vi "JTAG Clocks.vi"(0 "Adjust MCLK":bool, 1 "MCLK Source":u8(ring) items=["DCOCLK", "DCOCLK", "XT2CLK", "LFXT1/VLOCLK"], 2 "MCLK Divider":u8(ring) items=["1", "2", "4", "8"], 3 "Adjust SMCLK":bool, 4 "SMCLK Source":u8(ring) items=["DCOCLK", "XT2/LFXT1/VLOCLK"], 5 "SMCLK Divider":u8(ring) items=["1", "2", "4", "8"], 7 "error in (no error)":errorcluster, 8 "Adjust ACLK":bool, 9 "Adjust DCOCLK":bool, 10 "ACLK Source":u8(ring) items=["LFXT1CLK", "Reserved", "VLOCLK", "DIG EXT CLK"], 11 "DCO Range[0-15]":u8 max=15 step=1, 12 "ACLK Divider":u8(ring) items=["1", "2", "4", "8"], 13 "DCO Select[0-7]":u8 max=7 step=1, 15 "DCO Mod[0-31]":u8 max=31 step=1, 22 "DCO Ext. Res.":bool, 23 "LFXT1 XTS \"HI\"":bool, 24 "LFXT1 CAP":u8(ring)=1 items=["1pF", "6pF", "10pF", "12.5pF"], 25 "XT2 \"OFF\"":bool) -> (20 "LFXT1 Fault":bool, 21 "XT2 Fault":bool, 27 "error out":errorcluster)   [LabVIEW 2009]
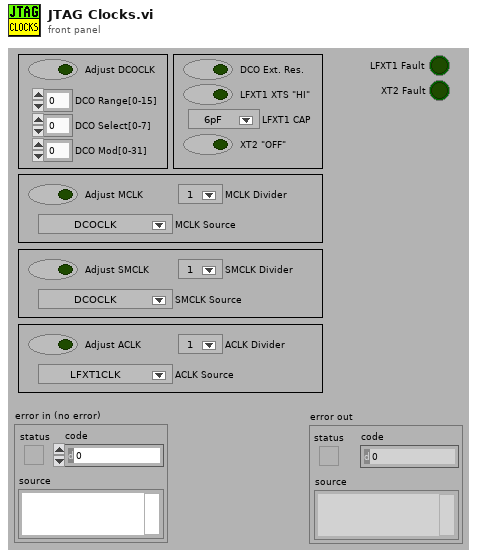
[diagram p1: front panel]
types:
  T1 = cluster{"ARG1-ARG7[0]":u16, "ARG1-ARG7[1]":u16, "ARG1-ARG7[2]":u16, "ARG1-ARG7[3]":u16, "ARG1-ARG7[4]":u16, "ARG1-ARG7[5]":u16, "ARG1-ARG7[6]":u16}
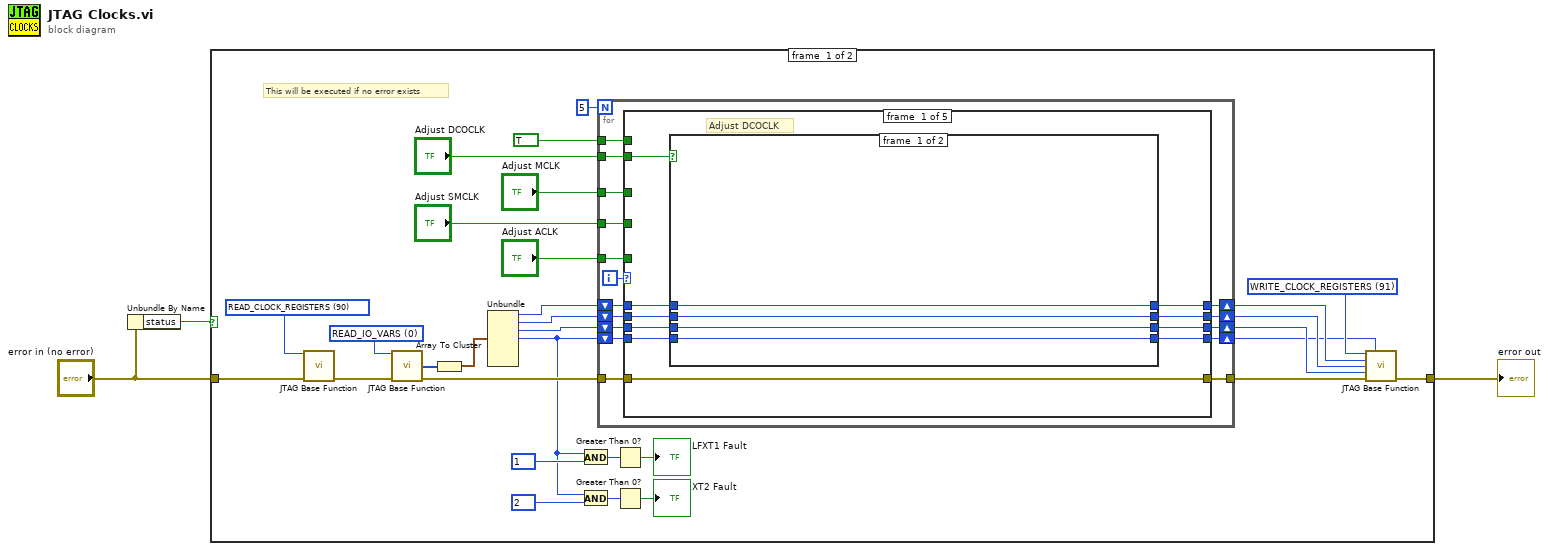
[diagram p0: block diagram]
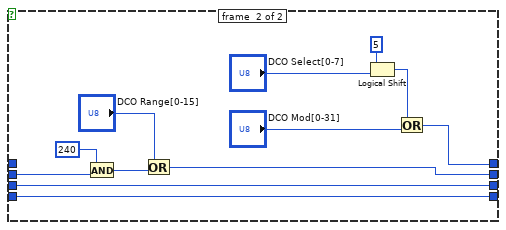
[diagram p2: hidden frame]
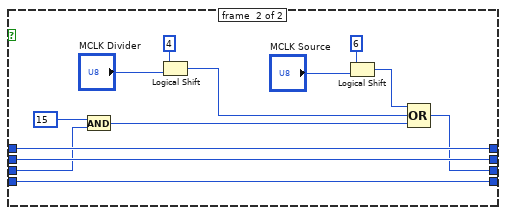
[diagram p4: hidden frame]
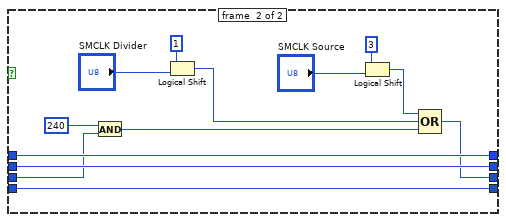
[diagram p6: hidden frame]
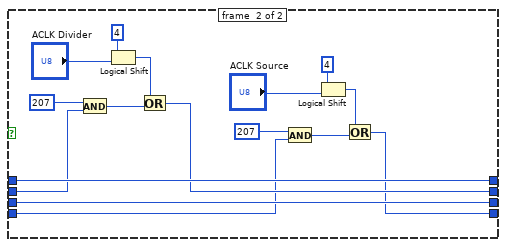
[diagram p8: hidden frame]
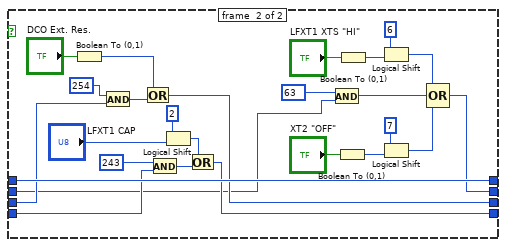
[diagram p10: hidden frame]
diagram:
  n1 = Unbundle By Name("error in (no error)") -> ("status"=w2:bool)
  n2 = case shown="False" w2 {
    tunnel: [w33 w200] -> w3
    tunnel: "error in (no error)" -> [w31 w200]
    frame #0 {
      w28 = u16 91 items=["READ_IO_VARS"=0, "PORT_OUT"=1, "PORT_SEL"=2, "PORT_REN"=3, "PORT_IN"=4, "PORT_DIR"=5, "SET_LCM"=6, "PWR_WRITE_SINGLE"=12, "PWR_READ_SINGLE"=13, "PWR_WRITE_MASK"=16, "PWR_WRITE_TRIM_DEFAULTS"=17, "STIM_POWER_UP"=20, "STIM_POWER_DN"=21, "STIM_WRITE_SINGLE"=22, "STIM_READ_SINGLE"=23, "STIM_WRITE_BLOCK"=24, "STIM_READ_BLOCK"=25, "STIM_WRITE_MASK"=26, "MICS_POWER_UP"=30, "MICS_POWER_DN"=31, "MICS_WRITE_SINGLE"=32, "MICS_READ_SINGLE"=33, "MICS_WRITE_BLOCK"=34, "MICS_READ_BLOCK"=35, "MICS_WRITE_MASK"=36, "MEM_POWER_UP"=40, "MEM_POWER_DN"=41, "MEM_WRITE_SINGLE"=42, "MEM_READ_SINGLE"=43, "MEM_WRITE_BLOCK"=44, "MEM_READ_BLOCK"=45, "MEM_WRITE_MASK"=46, "MEM_WRITE_SR"=47, "MEM_READ_SR"=48, "MEM_WRITE_OPCODE"=49, "INIT_PORTS"=50, "INIT_COMMS"=60, "RELEASE_COMMS"=61, "INIT_VARS"=62, "DCO_1MHZ"=63, "DCO_8MHZ"=64, "STANDARD_STARTUP"=65, "SET_LCM"=66, "PLUTO_WRITE_TRIM_DEFAULTS"=67, "SATURN_DIG_STARTUP"=68, "SATURN_BBC_STARTUP"=69, "SATURN_BBC_SHUTDOWN"=70, "START_STIM_CLK"=80, "STOP_STIM_CLK"=81, "PULSE_STIM_CLK"=82, "PULSE_STIM_SCK"=83, "SINGLE_ADC12"=85, "SINGLE_ADC12_REPEAT"=86, "MULTI_ADC12"=87, "MULTI_ADC12_REPEAT"=88, "DISABLE_ADC12"=89, "READ_CLOCK_REGISTERS"=90, "WRITE_CLOCK_REGISTERS"=91, "TC_STIM_RAM_READ"=200, "TC_STIM_RAM_WRITE"=201, "TC_TIMING_TEST"=220] ("Function")
      w29 = u16 0 items=["READ_IO_VARS"=0, "PORT_OUT"=1, "PORT_SEL"=2, "PORT_REN"=3, "PORT_IN"=4, "PORT_DIR"=5, "SET_LCM"=6, "PWR_WRITE_SINGLE"=12, "PWR_READ_SINGLE"=13, "PWR_WRITE_MASK"=16, "PWR_WRITE_TRIM_DEFAULTS"=17, "STIM_POWER_UP"=20, "STIM_POWER_DN"=21, "STIM_WRITE_SINGLE"=22, "STIM_READ_SINGLE"=23, "STIM_WRITE_BLOCK"=24, "STIM_READ_BLOCK"=25, "STIM_WRITE_MASK"=26, "MICS_POWER_UP"=30, "MICS_POWER_DN"=31, "MICS_WRITE_SINGLE"=32, "MICS_READ_SINGLE"=33, "MICS_WRITE_BLOCK"=34, "MICS_READ_BLOCK"=35, "MICS_WRITE_MASK"=36, "MEM_POWER_UP"=40, "MEM_POWER_DN"=41, "MEM_WRITE_SINGLE"=42, "MEM_READ_SINGLE"=43, "MEM_WRITE_BLOCK"=44, "MEM_READ_BLOCK"=45, "MEM_WRITE_MASK"=46, "MEM_WRITE_SR"=47, "MEM_READ_SR"=48, "MEM_WRITE_OPCODE"=49, "INIT_PORTS"=50, "INIT_COMMS"=60, "RELEASE_COMMS"=61, "INIT_VARS"=62, "DCO_1MHZ"=63, "DCO_8MHZ"=64, "STANDARD_STARTUP"=65, "SET_LCM"=66, "PLUTO_WRITE_TRIM_DEFAULTS"=67, "SATURN_DIG_STARTUP"=68, "SATURN_BBC_STARTUP"=69, "SATURN_BBC_SHUTDOWN"=70, "START_STIM_CLK"=80, "STOP_STIM_CLK"=81, "PULSE_STIM_CLK"=82, "PULSE_STIM_SCK"=83, "SINGLE_ADC12"=85, "SINGLE_ADC12_REPEAT"=86, "MULTI_ADC12"=87, "MULTI_ADC12_REPEAT"=88, "DISABLE_ADC12"=89, "READ_CLOCK_REGISTERS"=90, "WRITE_CLOCK_REGISTERS"=91, "TC_STIM_RAM_READ"=200, "TC_STIM_RAM_WRITE"=201, "TC_TIMING_TEST"=220] ("Function")
      w30 = u16 90 items=["READ_IO_VARS"=0, "PORT_OUT"=1, "PORT_SEL"=2, "PORT_REN"=3, "PORT_IN"=4, "PORT_DIR"=5, "SET_LCM"=6, "PWR_WRITE_SINGLE"=12, "PWR_READ_SINGLE"=13, "PWR_WRITE_MASK"=16, "PWR_WRITE_TRIM_DEFAULTS"=17, "STIM_POWER_UP"=20, "STIM_POWER_DN"=21, "STIM_WRITE_SINGLE"=22, "STIM_READ_SINGLE"=23, "STIM_WRITE_BLOCK"=24, "STIM_READ_BLOCK"=25, "STIM_WRITE_MASK"=26, "MICS_POWER_UP"=30, "MICS_POWER_DN"=31, "MICS_WRITE_SINGLE"=32, "MICS_READ_SINGLE"=33, "MICS_WRITE_BLOCK"=34, "MICS_READ_BLOCK"=35, "MICS_WRITE_MASK"=36, "MEM_POWER_UP"=40, "MEM_POWER_DN"=41, "MEM_WRITE_SINGLE"=42, "MEM_READ_SINGLE"=43, "MEM_WRITE_BLOCK"=44, "MEM_READ_BLOCK"=45, "MEM_WRITE_MASK"=46, "MEM_WRITE_SR"=47, "MEM_READ_SR"=48, "MEM_WRITE_OPCODE"=49, "INIT_PORTS"=50, "INIT_COMMS"=60, "RELEASE_COMMS"=61, "INIT_VARS"=62, "DCO_1MHZ"=63, "DCO_8MHZ"=64, "STANDARD_STARTUP"=65, "SET_LCM"=66, "PLUTO_WRITE_TRIM_DEFAULTS"=67, "SATURN_DIG_STARTUP"=68, "SATURN_BBC_STARTUP"=69, "SATURN_BBC_SHUTDOWN"=70, "START_STIM_CLK"=80, "STOP_STIM_CLK"=81, "PULSE_STIM_CLK"=82, "PULSE_STIM_SCK"=83, "SINGLE_ADC12"=85, "SINGLE_ADC12_REPEAT"=86, "MULTI_ADC12"=87, "MULTI_ADC12_REPEAT"=88, "DISABLE_ADC12"=89, "READ_CLOCK_REGISTERS"=90, "WRITE_CLOCK_REGISTERS"=91, "TC_STIM_RAM_READ"=200, "TC_STIM_RAM_WRITE"=201, "TC_TIMING_TEST"=220] ("Function")
      # "This will be executed if no error exists"
      n3 = call "JTAG Base Function.vi"("Function"=w30, "error in (no error)"=w31) -> ("error out"=w32:errorcluster)  [unwired: 11 in, 2 out]
      n4 = call "JTAG Base Function.vi"("Function"=w29, "error in (no error)"=w32) -> ("ARG1-ARG7"=w27:u16[], "error out"=w19:errorcluster)  [unwired: 11 in, 1 out]
      n5 = Array To Cluster(array=w27) -> (cluster=w26:T1)
      n6 = Unbundle(w26) -> ("ARG1-ARG7[0]"=w10:u16, "ARG1-ARG7[1]"=w11:u16, "ARG1-ARG7[2]"=w12:u16, "ARG1-ARG7[3]"=w13:u16)  [unwired: 3 out]
      n7 = And(x=w13, y=u8 1) -> (x .and. y?=w21:u16)
      n8 = And(x=w13, y=u8 2) -> (x .and. y?=w20:u16)
      n9 = for {
        N: 5 -> [_]
        tunnel: w19 -> [w49]
        tunnel: [w48] -> w18
        tunnel: "Adjust ACLK" -> [w46]
        tunnel: "Adjust SMCLK" -> [w45]
        tunnel: "Adjust MCLK" -> [w44]
        tunnel: "Adjust DCOCLK" -> [w43]
        shift-right: [w38] -> w6
        shift-left: w13 -> [w39]
        shift-right: [w37] -> w7
        shift-left: w12 -> [w40]
        shift-right: [w35] -> w8
        shift-left: w11 -> [w41]
        shift-right: [w36] -> w9
        shift-left: w10 -> [w42]
        tunnel: TRUE -> [w34]
        i -> [w47]
        n10 = case shown="2" w47 {
          tunnel: w49 -> [w59 w85 w112 w139 w169]
          tunnel: [w59 w85 w112 w139 w169] -> w48
          tunnel: w46 -> [_ _ _ w130 _]
          tunnel: w45 -> [_ _ w103 _ _]
          tunnel: w44 -> [_ w76 _ _ _]
          tunnel: w43 -> [w54 _ _ _ _]
          tunnel: w42 -> [w52 w79 w106 w133 w163]
          tunnel: w41 -> [w53 w80 w107 w134 w164]
          tunnel: w40 -> [w57 w83 w110 w137 w167]
          tunnel: w39 -> [w58 w84 w111 w138 w168]
          tunnel: [w55 w81 w108 w135 w165] -> w38
          tunnel: [w56 w82 w109 w136 w166] -> w37
          tunnel: [w51 w78 w105 w132 w162] -> w36
          tunnel: [w50 w77 w104 w131 w161] -> w35
          tunnel: w34 -> [_ _ _ _ w160]
          frame #0 {
            # "Adjust DCOCLK"
            n11 = case shown="True" w54 {
              tunnel: w58 -> [w60 w75]
              tunnel: w57 -> [w61 w74]
              tunnel: [w61 w74] -> w56
              tunnel: [w60 w75] -> w55
              tunnel: w53 -> [w62 w68]
              tunnel: w52 -> [w63 _]
              tunnel: [w63 w69] -> w51
              tunnel: [w62 w64] -> w50
              frame #0 {
              }
              frame #1 {
                n12 = And(x=u8 240, y=w68) -> (x .and. y?=w66:u16)
                n13 = Or(x="DCO Range[0-15]", y=w66) -> (x .or. y?=w64:u16)
                n14 = Logical Shift(y=i8 5, x="DCO Select[0-7]") -> (x << y=w71:u8)
                n15 = Or(x=w71, y="DCO Mod[0-31]") -> (x .or. y?=w69:u8)
              }
            }
          }
          frame #1 {
            # "Adjust MCLK"
            n16 = case shown="True" w76 {
              tunnel: w84 -> [w86 w102]
              tunnel: w83 -> [w87 w99]
              tunnel: [w87 w90] -> w82
              tunnel: [w86 w102] -> w81
              tunnel: w80 -> [w88 w100]
              tunnel: w79 -> [w89 w101]
              tunnel: [w89 w101] -> w78
              tunnel: [w88 w100] -> w77
              frame #0 {
              }
              frame #1 {
                n17 = And(x=u8 15, y=w99) -> (x .and. y?=w93:u16)
                n18 = Logical Shift(y=i8 4, x="MCLK Divider") -> (x << y=w91:u8)
                n19 = Logical Shift(y=i8 6, x="MCLK Source") -> (x << y=w92:u8)
                n20 = Compound Arithmetic op=OR(w92, w91, w93) -> (w90:u16)
              }
            }
          }
          frame #2 {
            # "Adjust SMCLK"
            n21 = case shown="True" w103 {
              tunnel: w111 -> [w113 w129]
              tunnel: w110 -> [w114 w124]
              tunnel: [w114 w123] -> w109
              tunnel: [w113 w129] -> w108
              tunnel: w107 -> [w115 w127]
              tunnel: w106 -> [w116 w128]
              tunnel: [w116 w128] -> w105
              tunnel: [w115 w127] -> w104
              frame #0 {
              }
              frame #1 {
                n22 = And(x=u8 240, y=w124) -> (x .and. y?=w125:u16)
                n23 = Logical Shift(y=i8 1, x="SMCLK Divider") -> (x << y=w118:u8)
                n24 = Logical Shift(y=i8 3, x="SMCLK Source") -> (x << y=w117:u8)
                n25 = Compound Arithmetic op=OR(w117, w118, w125) -> (w123:u16)
              }
            }
          }
          frame #3 {
            # "Adjust ACLK"
            n26 = case shown="True" w130 {
              tunnel: w138 -> [w140 w145]
              tunnel: w137 -> [w141 w159]
              tunnel: [w141 w159] -> w136
              tunnel: [w140 w144] -> w135
              tunnel: w134 -> [w142 w152]
              tunnel: w133 -> [w143 w158]
              tunnel: [w143 w158] -> w132
              tunnel: [w142 w151] -> w131
              frame #0 {
              }
              frame #1 {
                n27 = And(x=u8 207, y=w152) -> (x .and. y?=w154:u16)
                n28 = Logical Shift(y=i8 4, x="ACLK Divider") -> (x << y=w153:u8)
                n29 = Or(x=w153, y=w154) -> (x .or. y?=w151:u16)
                n30 = And(x=u8 207, y=w145) -> (x .and. y?=w149:u16)
                n31 = Logical Shift(y=i8 4, x="ACLK Source") -> (x << y=w146:u8)
                n32 = Or(x=w146, y=w149) -> (x .or. y?=w144:u16)
              }
            }
          }
          frame #4 {
            # "Adjust MISC"
            n33 = case shown="True" w160 {
              tunnel: w168 -> [w170 w193]
              tunnel: w167 -> [w171 w178]
              tunnel: [w171 w177] -> w166
              tunnel: [w170 w192] -> w165
              tunnel: w164 -> [w172 w174]
              tunnel: w163 -> [w173 w199]
              tunnel: [w173 w199] -> w162
              tunnel: [w172 w187] -> w161
              frame #0 {
              }
              frame #1 {
                n34 = Boolean To (0,1)(Boolean="DCO Ext. Res.") -> (0, 1=w188:i16)
                n35 = And(x=u8 254, y=w178) -> (x .and. y?=w190:u16)
                n36 = Or(x=w188, y=w190) -> (x .or. y?=w177:u16)
                n37 = And(x=u8 243, y=w193) -> (x .and. y?=w198:u16)
                n38 = Logical Shift(y=i8 2, x="LFXT1 CAP") -> (x << y=w196:u8)
                n39 = Or(x=w196, y=w198) -> (x .or. y?=w192:u16)
                n40 = And(x=u8 63, y=w174) -> (x .and. y?=w175:u16)
                n41 = Boolean To (0,1)(Boolean="XT2 \"OFF\"") -> (0, 1=w181:i16)
                n42 = Boolean To (0,1)(Boolean="LFXT1 XTS \"HI\"") -> (0, 1=w182:i16)
                n43 = Logical Shift(y=i8 6, x=w182) -> (x << y=w180:i16)
                n44 = Logical Shift(y=i8 7, x=w181) -> (x << y=w179:i16)
                n45 = Compound Arithmetic op=OR(w180, w175, w179) -> (w187:u16)
              }
            }
          }
        }
      }
      n46 = Greater Than 0?(x=w21) -> (x > 0?=→"LFXT1 Fault":bool)
      n47 = Greater Than 0?(x=w20) -> (x > 0?=→"XT2 Fault":bool)
      n48 = call "JTAG Base Function.vi"("Function"=w28, "ARG 4"=w6, "ARG 1"=w9, "ARG 2"=w8, "ARG 3"=w7, "error in (no error)"=w18) -> ("error out"=w33:errorcluster)  [unwired: 7 in, 2 out]
    }
    frame #1 {
      # "Error exists, skip all functions"
    }
  }
  "error out" <- w3
